vi "Get DVR for class path.vi"(0 "Class Path":path, 11 "Error In":errorcluster) -> (4 "DVR Out":refnum<data-value>, 15 "Error Out":errorcluster)   [LabVIEW 2020, in "Test.lvclass"]
uses:
  Test.lvclass
panel:
  out "Test out":refnum<class "Test.lvclass">
  in  "Test in":refnum<class "Test.lvclass">
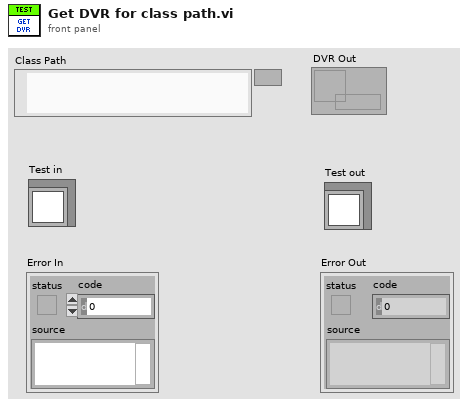
[diagram p1: front panel]
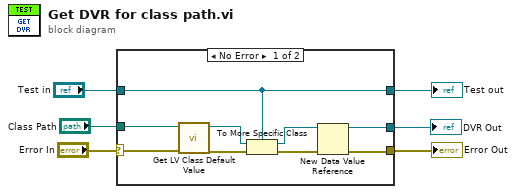
[diagram p0: block diagram]
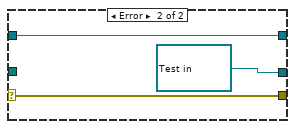
[diagram p2: hidden frame]
diagram:
  n1 = case shown="No Error" "Error In" {
    selector: "Error In" -> [w15 w18]
    tunnel: [w8 w18] -> w5
    tunnel: [w11 w17] -> w3
    tunnel: "Test in" -> [w11 w17]
    tunnel: "Class Path" -> [w14 _]
    tunnel: [w7 refnum<data-value> refnum ("data value reference")] -> w1
    frame No Error {
      n2 = call <vilib>:"Get LV Class Default Value.vi"("error in (no error)"=w15, "class path"=w14) -> ("error out"=w13:errorcluster, "object"=w12:refnum<class>)  [unwired: 8 in]
      n3 = To More Specific Class(target class=w11, reference=w12, error in=w13) -> (specific class reference=w9:refnum<class "Test.lvclass">, error out=w10:errorcluster)
      n4 = New Data Value Reference(data value=w9, error in=w10) -> (data value reference=w7:refnum<data-value>, error out=w8:errorcluster)
    }
    frame Error {
    }
  }
  "Error Out" <- w5
  "Test out" <- w3
  "DVR Out" <- w1
